vi "Write DataGridViewNet.vi"(8 "error in (no error)":errorcluster, 10 "DataGridView":refnum<k24>, 11 "datagrid in":refnum<class "Data Grid.lvclass">) -> (0 "error out":errorcluster, 3 "datagrid out":refnum<class "Data Grid.lvclass">)   [LabVIEW 2013, in "Table Manager.lvlib" / "Data Grid.lvclass"]
uses:
  Data Grid.lvclass
  System.Windows.Forms
  Data Grid.lvclass/Data Grid.ctl
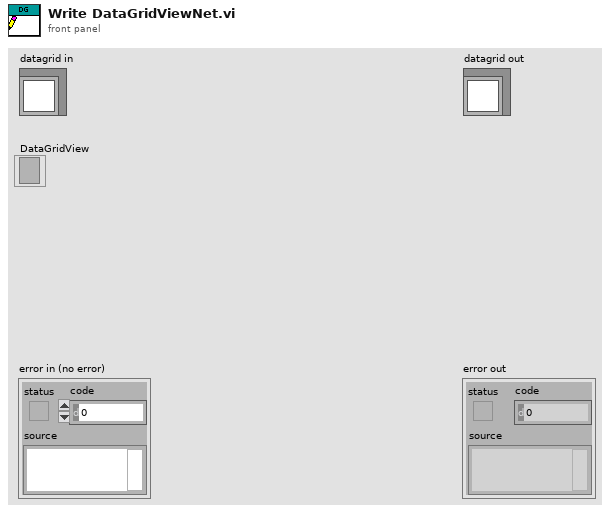
[diagram p1: front panel]
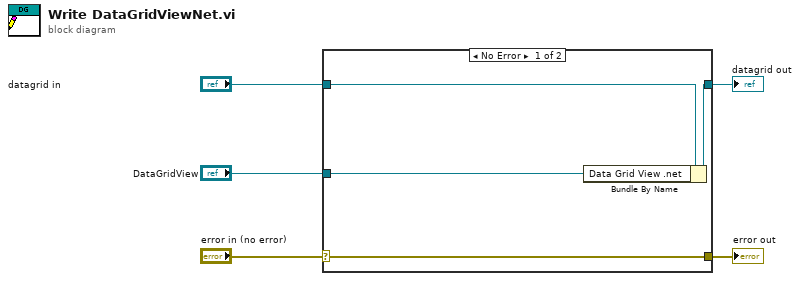
[diagram p0: block diagram]
diagram:
  n1 = case shown="No Error" "error in (no error)" {
    selector: "error in (no error)" -> [w9 w10]
    tunnel: [w9 w10] -> w4
    tunnel: [w7 w11] -> w2
    tunnel: "datagrid in" -> [w8 w11]
    tunnel: "DataGridView" -> [w6 _]
    frame No Error {
      n2 = Bundle By Name(cluster=w8, "Data Grid View .net"=w6) -> (w7:refnum<class "Data Grid.lvclass">)
    }
    frame Error {
    }
  }
  "error out" <- w4
  "datagrid out" <- w2
